vi "ShiftKeySetting.vi"(10 "Shift key behaviour":T1, 11 "Shift pressed?":bool) -> (3 "Terminals only?":bool)   [LabVIEW 2017, in "ErrorStructureDrawer.lvlib"]
doc: "Returns boolean to indicate whether the plugin should only handle error terminals (true state). False means the full plugin functionality should be carried out - i.e. creation of an error structure."
uses:
  ErrorStructureDrawer.lvlib
  Controls/ShiftKeyBehaviour.ctl
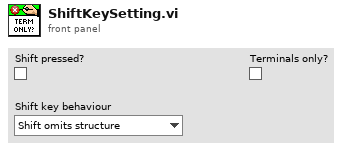
[diagram p1: front panel]
types:
  T1 = typedef "ErrorStructureDrawer.lvlib/ShiftKeyBehaviour.ctl" = enum16{"Shift omits structure", "Shift includes structure"}
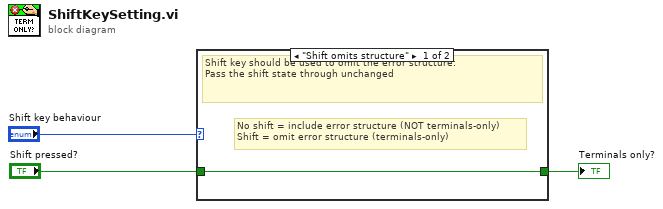
[diagram p0: block diagram]
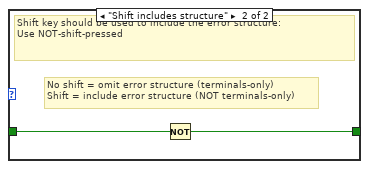
[diagram p2: hidden frame]
diagram:
  n1 = case shown="\"Shift omits structure\"" "Shift key behaviour" {
    tunnel: "Shift pressed?" -> [w4 w6]
    tunnel: [w4 w5] -> w2
    frame "Shift omits structure" {
      # "No shift = include error structure (NOT terminals-only)\nShift = omit error structure (terminals-only)"
      # "Shift key should be used to omit the error structure:\nPass the shift state through unchanged"
    }
    frame "Shift includes structure" {
      # "No shift = omit error structure (terminals-only)\nShift = include error structure (NOT terminals-only)"
      # "Shift key should be used to include the error structure:\nUse NOT-shift-pressed"
      n2 = Not(x=w6) -> (.not. x?=w5:bool)
    }
  }
  "Terminals only?" <- w2
